vi "RT init FAST.vi"() -> (1 "error out":errorcluster)   [LabVIEW 2012]
uses:
  FAST_RT_DLL.dll
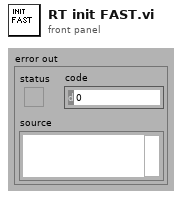
[diagram p1: front panel]
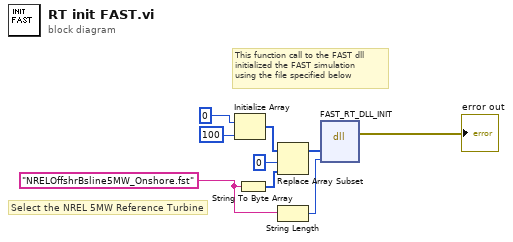
[diagram p0: block diagram]
diagram:
  w9 = "NRELOffshrBsline5MW_Onshore.fst"
  # "Select the NREL 5MW Reference Turbine"
  # "This function call to the FAST dll\ninitialized the FAST simulation\nusing the file specified below"
  n1 = Initialize Array(u8 0 ("element"), 100 ("dimension size")) -> (w5:u8[])
  n2 = String To Byte Array(string=w9) -> (unsigned byte array=w3:u8[])
  n3 = Replace Array Subset(array=w5, new element=w3, index=0) -> (w2:u8[])
  n4 = String Length(string=w9) -> (length=w8:i32)
  n5 = dll-call lib="C:/Users/MMonroe/Desktop/Current Opps/FAST RT DLL/demoVI_V8/FAST_RT_DLL.dll" fn="FAST_RT_DLL_INIT"("FileName"=w2, "FileLength"=w8) -> (error out=→"error out":errorcluster)  [unwired: 3 in, 4 out]
